vi "Handle GET logs.vi"(8 "error in (no error)":errorcluster, 10 "Response":refnum<class "Response.lvclass">, 11 "Request in":refnum<class "Request.lvclass">) -> (0 "error out":errorcluster, 2 "Handled?":bool)   [LabVIEW 2023, in "Server.lvclass"]
uses:
  Server.lvclass
  Response/Response.lvclass
  Request/Request.lvclass
  Request/Get Request.vi
  Server.lvclass/Server.ctl
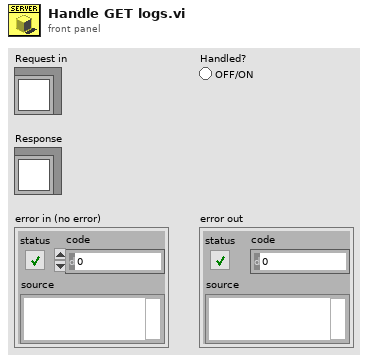
[diagram p1: front panel]
types:
  T1 = typedef "Request.ctl" = cluster{"Method":string, "URI":string, "Protocol":string, "Raw Path":string, "Query":string, "Fragment":string, "Raw Body":string, "Headers":variant, "Parameters":variant, "Body":variant, "Raw Header":string, "Path":string[]}
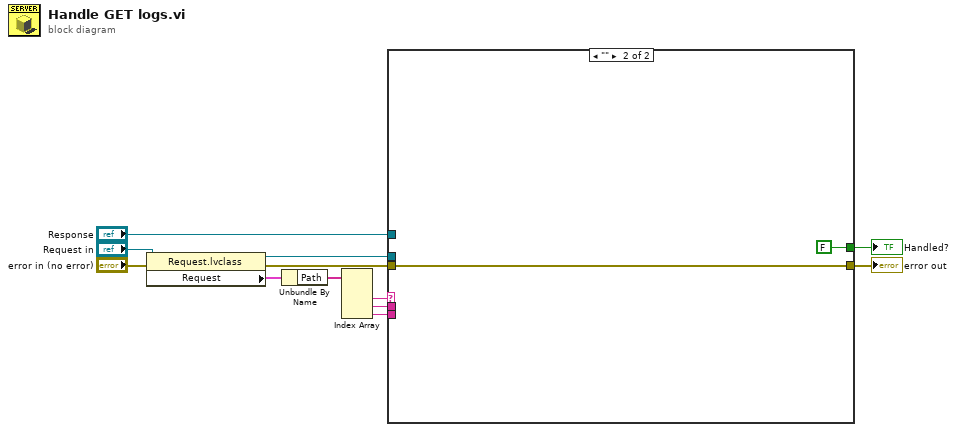
[diagram p0: block diagram]
diagram:
  n1 = property class="Request.lvclass"(reference="Request in", error in="error in (no error)") -> (reference out=w7:refnum<class "Request.lvclass">, error out=w8:errorcluster, "Request"=w5:T1)
  n2 = Unbundle By Name(w5) -> ("Path"=w4:string[])
  n3 = Index Array(array=w4) -> (element #2=w3:string, element #3=w2:string, element #4=w1:string)  [unwired: 4 in, 1 out]
  n4 = case shown="\"\"" w3 {
    tunnel: [_ FALSE] -> w9
    tunnel: w8 -> [w13 w14]
    tunnel: [w13 w14] -> w11
    tunnel: "Response" -> [_ _]
    tunnel: w7 -> [_ _]
    tunnel: w2 -> [_ _]
    tunnel: w1 -> [_ _]
    frame Default {
    }
    frame "" {
    }
  }
  "error out" <- w11
  "Handled?" <- w9
